vi "Initialize.vi"(6 "libssh2 Shared Library":path=path "", 8 "Error In":errorcluster, 11 "Flags":i32) -> (0 "Error Out":errorcluster)   [LabVIEW 2017, in "LabSSH2.lvlib"]
uses:
  LabSSH2.lvlib
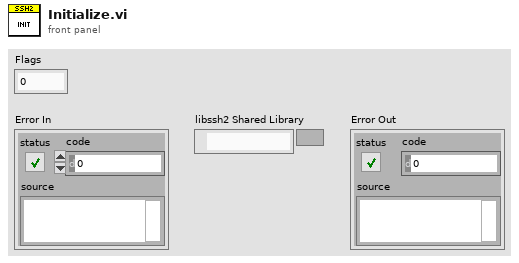
[diagram p1: front panel]
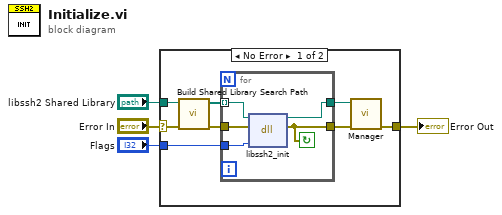
[diagram p0: block diagram]
diagram:
  n1 = case shown="No Error" "Error In" {
    selector: "Error In" -> [w10 w18]
    tunnel: "libssh2 Shared Library" -> [w9 _]
    tunnel: "Flags" -> [w8 _]
    tunnel: [w5 w18] -> w1
    frame No Error {
      n2 = call "Build Shared Library Search Path.vi"("Error In"=w10, "libssh2 Shared Library"=w9) -> ("Error Out"=w11:errorcluster, "Search Path"=w12:path[])  [unwired: 8 in]
      n3 = for {
        tunnel: w12 -> [w13] mode=indexing
        tunnel: w11 -> [w17]
        tunnel: [w16] -> w6
        tunnel: [w15] -> w7
        tunnel: w8 -> [w14]
        stop <- w15 continue-if-true
        n4 = dll-call lib="C:/Program Files/libssh2/bin/libssh2.dll" fn="libssh2_init"(path in=w13, error in=w17, "flags"=w14) -> (path out=w16:path, error out=w15:errorcluster)  [unwired: 3 in]
      }
      n5 = call "Manager.vi"("Error In"=w7, "Shared Library In"=w6) -> ("Error Out"=w5:errorcluster)  [unwired: 8 in, 1 out]
    }
    frame Error {
    }
  }
  "Error Out" <- w1
